vi "Feeder Control.vi"(4 "Collect from Feeder?":bool) -> ()   [LabVIEW 2012]
uses:
  BotStatus.vi
  Motors Values.vi
panel:
  out "Feeder Mode Enabled in Stack":bool
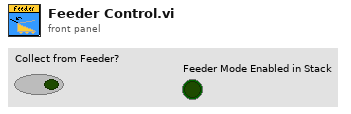
[diagram p1: front panel]
types:
  T1 = typedef "WPI_ServoDeviceRef.ctl" = cluster{"DeviceStatus":errorcluster, "Digital Module":T2, "PWM Channel":T3, "DeadBand":T4}
  T2 = typedef "FPGA_TypedefDigitalModule.ctl" = enum16{"Digital Module 1", "Digital Module 2"}
  T3 = typedef "FPGA_DIOPWMChannel.ctl" = enum8{"PWM 1", "PWM 2", "PWM 3", "PWM 4", "PWM 5", "PWM 6", "PWM 7", "PWM 8", "PWM 9", "PWM 10", "Invalid"}
  T4 = typedef "WPI_PWMDeadband.ctl" = cluster{"Name":string, "maxPositivePwm":i32, "minPositivePwm":i32, "centerPwm":i32, "maxNegativePwm":i32, "minNegativePwm":i32, "angularRange":u16}
  T5 = typedef "WPI_DigitalInputDevRef.ctl" = cluster{"DevStatus":errorcluster, "DIO Channel":T6, "Digital Module":T2}
  T6 = typedef "FPGA_DIOChannel.ctl" = enum8{"DIO 1", "DIO 2", "DIO 3", "DIO 4", "DIO 5", "DIO 6", "DIO 7", "DIO 8", "DIO 9", "DIO 10", "DIO 11", "DIO 12", "DIO 13", "DIO 14", "Invalid"}
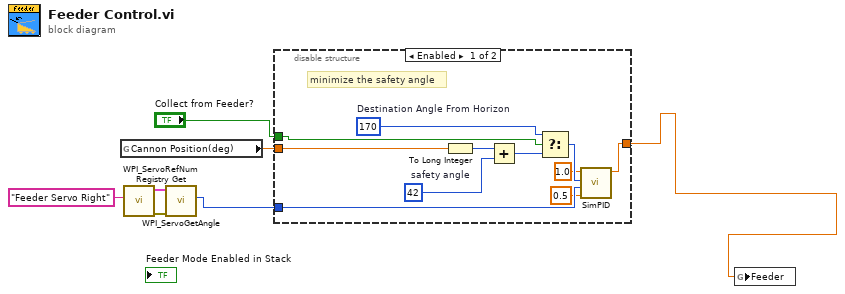
[diagram p0: block diagram]
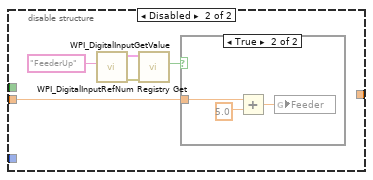
[diagram p2: hidden frame]
diagram:
  n1 = global read "BotStatus.vi" "Cannon Position(deg)"() -> (w7:dbl)
  n2 = call <vilib>:"WPI_ServoRefNum Registry Get.vi"("refnum name"="Feeder Servo Right") -> ("error out"=w4:errorcluster, "ServoDeviceRef"=w5:T1)  [unwired: 9 in]
  n3 = call <vilib>:"WPI_ServoGetAngle.vi"("ServoDeviceRef"=w5, "error in (no error)"=w4) -> ("Angle"=w2:u16)  [unwired: 6 in, 2 out]
  n4 = disable-structure shown="Enabled" {
    disable-tunnel: w7 -> [w17 w19]
    disable-tunnel: "Collect from Feeder?" -> [w15 _]
    disable-tunnel: [w11 _] -> w1
    disable-tunnel: w2 -> [w10 _]
    frame Enabled {
      w14 = 170  # Destination Angle From Horizon
      w18 = 42  # safety angle
      # "minimize the safety angle"
      n5 = To Long Integer(number=w17) -> (32bit integer=w13:i32)
      n6 = Add(x=w13, y=w18) -> (x+y=w16:i32)
      n7 = Select(t=w14, s=w15, f=w16) -> (s? t:f=w12:i32)
      n8 = call "SimPID.vi"("Range"=0.5, "Position"=w10, "Set Point"=w12, "Gain"=1.0) -> ("result"=w11:dbl)  [unwired: 5 in, 1 out]
    }
    frame Disabled {
      n9 = call <vilib>:"WPI_DigitalInputRefNum Registry Get.vi"("refnum name"="FeederUp") -> ("error out"=w21:errorcluster, "DigitalInputDevRef"=w20:T5)  [unwired: 9 in]
      n10 = call <vilib>:"WPI_DigitalInputGetValue.vi"("error in (no error)"=w21, "DigitalInputDevRef"=w20) -> ("Value"=w23:bool)  [unwired: 7 in, 2 out]
      n11 = case shown="True" w23 {
        tunnel: w19 -> [_ w26]
        frame False {
        }
        frame True {
          n12 = Add(x=w26, y=5.0) -> (x+y=w24:dbl)
          n13 = global write "Motors Values.vi" "Feeder"(w24) -> ()
        }
      }
    }
  }
  n14 = global write "BotStatus.vi" "Feeder"(w1) -> ()
